vi "Display Winning Score.vi"(11 "Game Board in":refnum<class "Game Board.lvclass">) -> ()   [LabVIEW 2021, in "Game Board.lvclass"]
doc: "MIT Licence\nCopyright (c) 2024 David Grollier"
uses:
  Game Board.lvclass
  Game Board.lvclass/Game Board.ctl
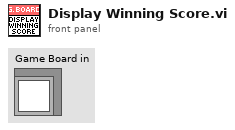
[diagram p1: front panel]
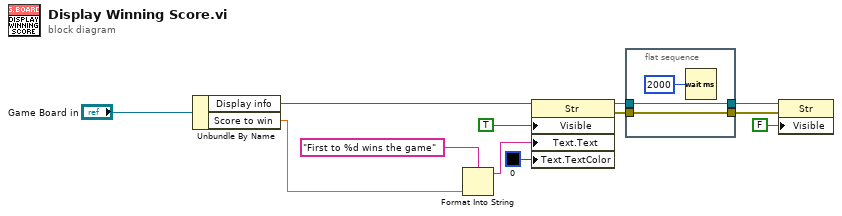
[diagram p0: block diagram]
diagram:
  n1 = Unbundle By Name("Game Board in") -> ("Display info"=w8:refnum<vi>, "Score to win"=w7:dbl)
  n2 = Format Into String(format string="First to %d wins the game", w7) -> (resulting string=w12:string)  [unwired: 2 in, 1 out]
  n3 = property class="Str"(reference=w8, "Visible"=TRUE, "Text.Text"=w12, "Text.TextColor"=u32 0 ("Text.Text Colors:Text Color")) -> (reference out=w6:refnum<vi>, error out=w3:errorcluster)  [unwired: 1 in]
  n4 = flat-sequence {
    tunnel: w6 -> [w15]
    tunnel: [w15] -> w5
    tunnel: w3 -> [w13]
    tunnel: [w13] -> w2
    frame #0 {
      n5 = Wait (ms)(milliseconds to wait=u32 2000) -> ()  [unwired: 1 out]
    }
  }
  n6 = property class="Str"(reference=w5, error in=w2, "Visible"=FALSE) -> ()  [unwired: 2 out]
